vi "xetCommandConnectionID.vi"(0 "Connection ID In":refnum<k5>, 1 "Get/Set":enum16{"Get", "Set"}(ring)) -> (3 "Connection ID Out":refnum<k5>, 4 "New Connection":bool, 5 "error out":errorcluster)   [LabVIEW 2016, in "h.Library.lvlib"]
uses:
  h.Library.lvlib
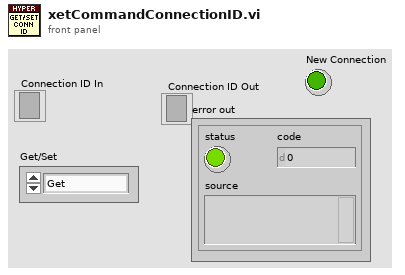
[diagram p1: front panel]
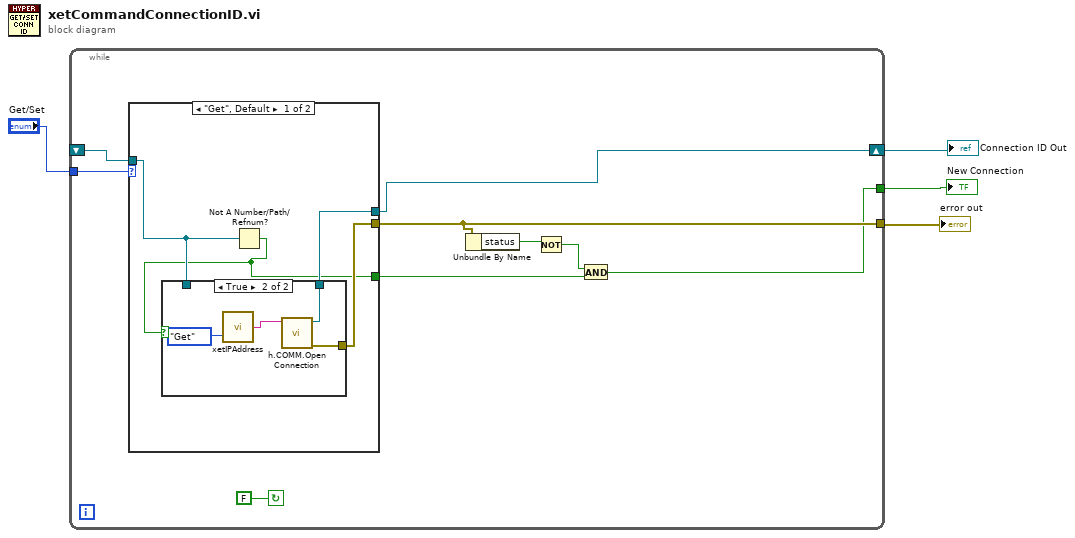
[diagram p0: block diagram]
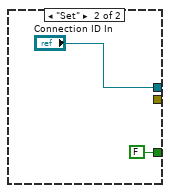
[diagram p3: hidden frame]
diagram:
  n1 = while {
    tunnel: "Get/Set" -> [w13]
    shift-right: [w10] -> w3
    shift-left: _ -> [w11]
    tunnel: [w8] -> w2
    tunnel: [w5] -> w1
    stop <- FALSE continue-if-true
    n2 = case shown="\"Get\", Default" w13 {
      tunnel: [w17 "Connection ID In"] -> w10
      tunnel: w11 -> [w15 _]
      tunnel: [w16 _] -> w8
      tunnel: [w14 FALSE] -> w9
      frame "Get", Default {
        n3 = Not A Number/Path/Refnum?(number/path/refnum=w15) -> (NaN/Path/Refnum?=w14:bool)
        n4 = case shown="True" w14 {
          tunnel: [w18 w20] -> w17
          tunnel: [_ w19] -> w16
          tunnel: w15 -> [w18 _]
          frame False {
          }
          frame True {
            n5 = call "xetIPAddress.vi"("Get/Set"=enum16{"Get", "Set"}."Get") -> ("IP Address Out"=w21:string)  [unwired: 1 in]
            n6 = call "h.COMM.Open Connection.vi"("Address"=w21) -> ("error out"=w19:errorcluster, "Connection ID"=w20:refnum<k5>)  [unwired: 9 in]
          }
        }
      }
      frame "Set" {
      }
    }
    n7 = Unbundle By Name(w8) -> ("status"=w7:bool)
    n8 = Not(x=w7) -> (.not. x?=w6:bool)
    n9 = And(x=w6, y=w9) -> (x .and. y?=w5:bool)
  }
  "Connection ID Out" <- w3
  "error out" <- w2
  "New Connection" <- w1
